vi "RequestInsertEvents_dir.vi"(5 "Events":T1[](array[typedef]), 11 "error in (no error)":errorcluster) -> (6 "request":string, 15 "error out":errorcluster)   [LabVIEW 2019, in "Logger.lvclass"]
uses:
  Logger.lvclass
  EventData.ctl
  EventCode.ctl
  Priority.ctl
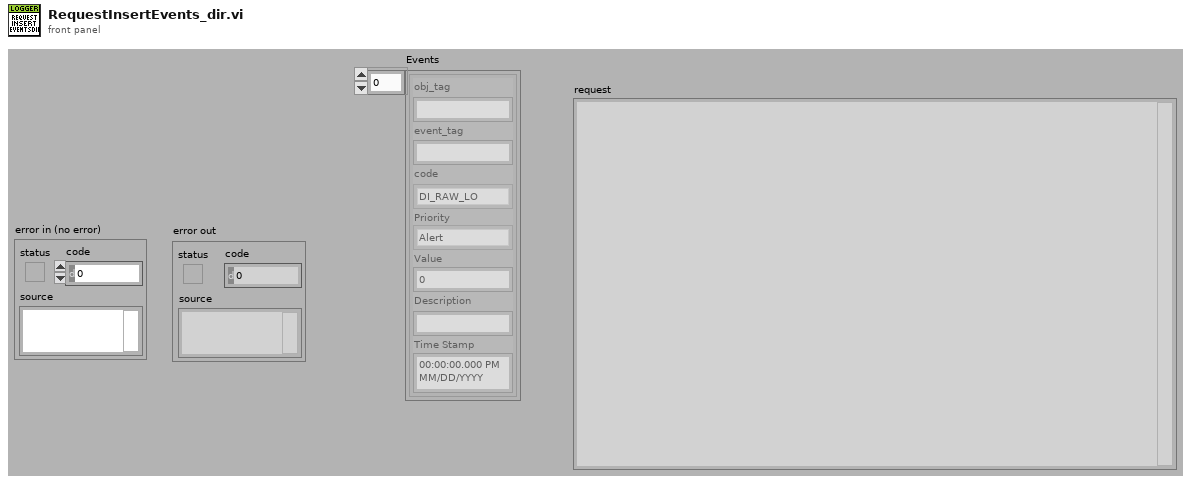
[diagram p1: front panel]
types:
  T1 = typedef "Logger.lvclass/EventData.ctl" = cluster{"obj_tag":string, "event_tag":string, "code":T2, "Priority":T3, "Value":dbl, "Description":string, "Time Stamp":timestamp}
  T2 = typedef "Logger.lvclass/EventCode.ctl" = enum16{"DI_EU_LO", "DI_EU_HI", "DIO_LO", "DIO_HI", "DI_RAW_LO", "DI_RAW_HI", "DO_LO", "DO_HI", "DA_OK", "DA_ALARM", "AA_HI", "AA_HIHI", "AA_LO", "AA_LOLO", "AA_OK", "CMD", "OUT_OF_RANGE_OK", "OUT_OF_RANGE_LO", "OUT_OF_RANGE_HI", "CONFIG", "DI_LO", "DI_HI"}
  T3 = typedef "Logger.lvclass/Priority.ctl" = enum16{"Alert", "Critical", "Error", "Warning", "Notice", "Informational", "Debug"}
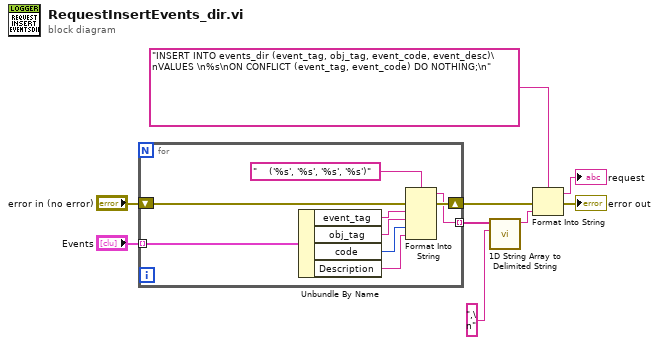
[diagram p0: block diagram]
diagram:
  n1 = for {
    tunnel: [w17] -> w8 mode=indexing
    tunnel: "Events" -> [w14] mode=indexing
    shift-right: [w18] -> w3
    shift-left: "error in (no error)" -> [w16]
    n2 = Unbundle By Name(w14) -> ("event_tag"=w13:string, "obj_tag"=w12:string, "code"=w11:T2, "Description"=w10:string)
    n3 = Format Into String(format string="    ('%s', '%s', '%s', '%s')", error in=w16, w13, w12, w11, w10) -> (resulting string=w17:string, error out=w18:errorcluster)  [unwired: 1 in]
  }
  n4 = call <vilib>:"1D String Array to Delimited String.vi"("delimiter"=",\n", "string array"=w8) -> ("delimited string"=w4:string)  [unwired: 9 in]
  n5 = Format Into String(format string="INSERT INTO events_dir (event_tag, obj_tag, event_code, event_desc)\nVALUES \n%s\nON CONFLICT (event_tag, event_code) DO NOTHING;\n", error in=w3, w4) -> (resulting string=→"request":string, error out=→"error out":errorcluster)  [unwired: 1 in]
